vi "PSCHN_Update Tree.vi"(8 "error in (no error)":errorcluster, 9 "Cards":T1[](array[typedef]), 10 "PopUp Para":T3, 11 "Tree":refnum<vi>) -> (0 "error out":errorcluster)   [LabVIEW 2016]
uses:
  Controls/PSCHN_Card Para.ctl
  Controls/PSCHN_Channel Para.ctl
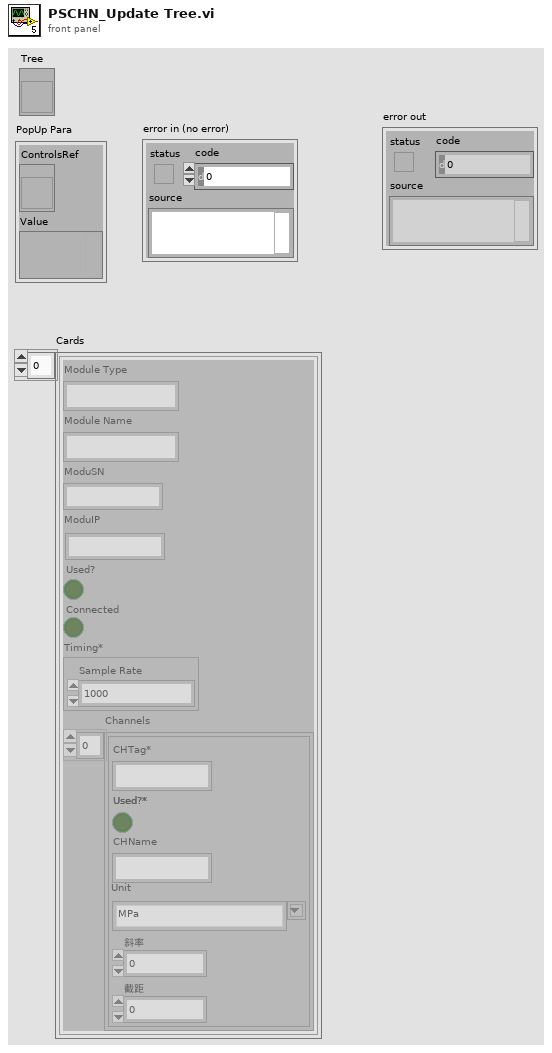
[diagram p1: front panel]
types:
  T1 = typedef "PSCHN_Card Para.ctl" = cluster{"Module Type":string, "Module Name":string, "ModuSN":string, "ModuIP":string, "Used?":bool, "Connected":bool, "Timing*":cluster{"Sample Rate":dbl}, "Channels":T2[]}
  T2 = typedef "PSCHN_Channel Para.ctl" = cluster{"CHTag*":string, "Used?*":bool, "CHName":string, "Unit":string, "斜率":dbl, "截距":dbl}
  T3 = cluster{"ControlsRef":refnum<vi>, "Value":variant}
  T4 = cluster{"Left Cell String":string, "Child Text":string[], "Child Tag":string, "Item Indent":i32, "Child Only?":bool, "Glyph Index":i32}
  T5 = typedef "PSCFO_ParaDataType.ctl" = cluster{"ParaTag":string, "ParaName":string, "ParaType":string, "PicName":string, "ParaLevel":string, "DefaultValue":variant, "ParaVisable?":bool, "ParaOperation?":bool, "Operation":cluster{"ParaValue":string, "Operation":cluster{"ChangePara":cluster{"ParaName":string, "ParaData":string}[], "EnablePara":string[]}}[], "Ring Para":T6}
  T6 = typedef "PSLIST_Para Related.ctl" = cluster{"Strings":string[], "Values":ext[], "Use":bool, "Combox":string[], "Browse Options":T7, "Combo Box":cluster{"Allow Undefined Strings":bool}}
  T7 = typedef "LVBrowseOptionsTypeDef.ctl" = cluster{"Prompt":string, "Match Pattern":string, "Mode":enum32{"existing file", "new file", "new or existing file", "existing dir", "new dir", "new or existing dir", "existing file (use LLBs)", "new file (use LLBs)", "new or existing file (use LLBs)", "new or existing file or directory (use LLBs)", "existing dir (use LLBs)", "new dir (use LLBs)", "new or existing dir (use LLBs)", "existing file or dir", "new file or dir", "new or existing file or dir", "existing file or dir (use LLBs)", "new file or dir (use LLBs)"}, "Start Path":path, "Pattern Label":string, "Button Text":string}
  T8 = cluster{"Left Cell String":string, "Child Text":string[], "Child Tag":string, "Item Indent":i32, "Child Only?":bool, "Glyph Index":i32}[]
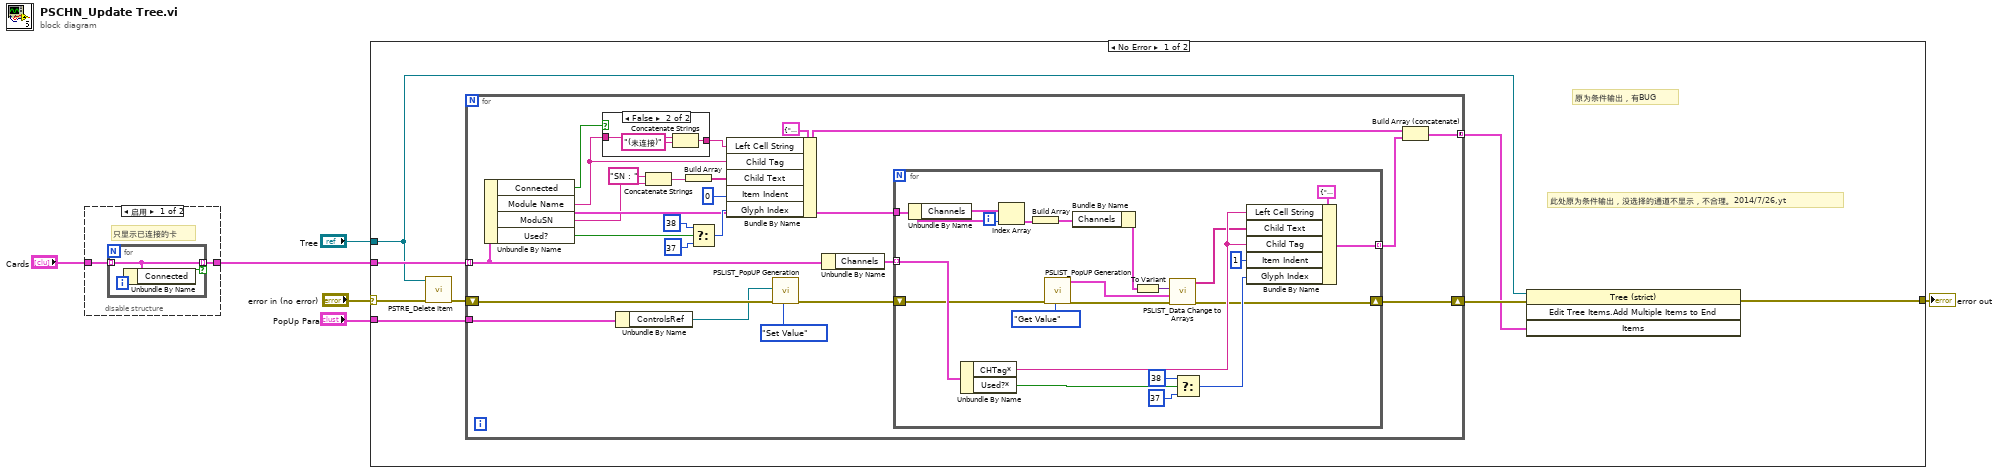
[diagram p0: block diagram]
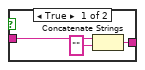
[diagram p3: hidden frame]
diagram:
  n1 = disable-structure shown="启用" {
    disable-tunnel: "Cards" -> [w8 w11]
    disable-tunnel: [w7 w11] -> w1
    frame Enabled {
      # "只显示已连接的卡"
      n2 = for {
        tunnel: w8 -> [w10] mode=indexing
        tunnel: [w10] -> w7 mode=indexing if=w9
        n3 = Unbundle By Name(w10) -> ("Connected"=w9:bool)
      }
    }
    frame Disabled {
    }
  }
  n4 = case shown="No Error" "error in (no error)" {
    selector: "error in (no error)" -> [w17 w72]
    tunnel: [w18 w72] -> w6
    tunnel: w1 -> [w15 _]
    tunnel: "Tree" -> [w13 _]
    tunnel: "PopUp Para" -> [w12 _]
    frame No Error {
      # "此处原为条件输出，没选择的通道不显示，不合理。2014/7/26,yt"
      # "原为条件输出，有BUG"
      n5 = call <vilib>:"PSTRE_Delete Item.vi"("error in"=w17, "Tree Ref"=w13) -> ("error out"=w16:errorcluster)  [unwired: 8 in, 1 out]
      n6 = for {
        tunnel: w15 -> [w34] mode=indexing
        shift-right: [w43] -> w19
        shift-left: w16 -> [w32]
        tunnel: [w36] -> w14 mode=concatenating
        tunnel: w12 -> [w33]
        n7 = Unbundle By Name(w34) -> ("Connected"=w28:bool, "Module Name"=w27:string, "ModuSN"=w23:string, "Used?"=w24:bool)
        n8 = case shown="False" w28 {
          tunnel: w27 -> [w46 w49]
          tunnel: [w45 w48] -> w26
          frame True {
            n9 = Concatenate Strings(w46, "" ("字符串")) -> (w45:string)
          }
          frame False {
            n10 = Concatenate Strings(w49, "(未连接)" ("字符串")) -> (w48:string)
          }
        }
        n11 = Unbundle By Name(w33) -> ("ControlsRef"=w30:refnum<vi>)
        n12 = Concatenate Strings("SN : " ("字符串"), w23) -> (w21:string)
        n13 = Build Array(w21) -> (w20:string[])
        n14 = Select(t=38 ("symbol (no symbol=0)"), s=w24, f=37 ("symbol (no symbol=0)")) -> (s? t:f=w39:i32)
        n15 = Bundle By Name(cluster=T4 {"Left Cell String"="", "Child Text"=[], "Child Tag"="", "Item Indent"=0, "Child Only?"=FALSE, "Glyph Index"=0} ("t"), "Left Cell String"=w26, "Child Tag"=w27, "Child Text"=w20, "Item Indent"=0, "Glyph Index"=w39) -> (w38:T4)
        n16 = call <vilib>:"PSLIST_PopUP Generation.vi"("Commond"=enum16{"Set Value", "Get Value"}."Set Value", "错误输入（无错误）"=w32, "ControlsRef"=w30) -> ("error out"=w31:errorcluster)  [unwired: 7 in, 1 out]
        n17 = Unbundle By Name(w34) -> ("Channels"=w35:T2[])
        n18 = for {
          shift-right: [w52] -> w43
          shift-left: w31 -> [w55]
          tunnel: w35 -> [w63] mode=indexing
          tunnel: w34 -> [w65]
          tunnel: [w61] -> w37 mode=indexing
          i -> [w67]
          n19 = Unbundle By Name(w65) -> ("Channels"=w68:T2[])
          n20 = Unbundle By Name(w63) -> ("CHTag*"=w58:string, "Used?*"=w69:bool)
          n21 = Index Array(array=w68, index=w67) -> (element=w66:T2)
          n22 = Build Array(w66) -> (w64:T2[])
          n23 = call <vilib>:"PSLIST_PopUP Generation.vi"("Commond"=enum16{"Set Value", "Get Value"}."Get Value", "错误输入（无错误）"=w55) -> ("error out"=w56:errorcluster, "PopUpPara"=w51:T5[])  [unwired: 8 in]
          n24 = Bundle By Name(cluster=w65, "Channels"=w64) -> (w54:T1)
          n25 = To Variant(anything=w54) -> (Variant=w53:variant)
          n26 = call <vilib>:"PSLIST_Data Change to Arrays.vi"("Error In"=w56, "Parameter"=w51, "VData"=w53) -> ("Error Out"=w52:errorcluster, "Values"=w50:string[])  [unwired: 7 in]
          n27 = Select(t=38 ("symbol (no symbol=0)"), s=w69, f=37 ("symbol (no symbol=0)")) -> (s? t:f=w59:i32)
          n28 = Bundle By Name(cluster=T4 {"Left Cell String"="", "Child Text"=[], "Child Tag"="", "Item Indent"=0, "Child Only?"=FALSE, "Glyph Index"=0} ("t"), "Left Cell String"=w58, "Child Text"=w50, "Child Tag"=w58, "Item Indent"=1, "Glyph Index"=w59) -> (w61:T4)
        }
        n29 = Build Array (concatenate)(w38, w37) -> (w36:T8)
      }
      n30 = invoke class="Tree (strict)" method="Edit Tree Items.Add Multiple Items to End"(reference=w13, error in=w19, "Items"=w14) -> (error out=w18:errorcluster)  [unwired: 1 in, 3 out]
    }
    frame Error {
    }
  }
  "error out" <- w6
